vi "Distance Regression Calc.vi"(10 "Numeric in":i32, 11 "Y":dbl) -> (3 "Distance":ext)   [LabVIEW 2025]
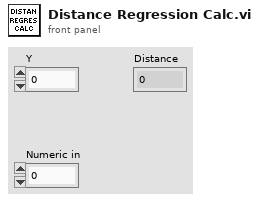
[diagram p1: front panel]
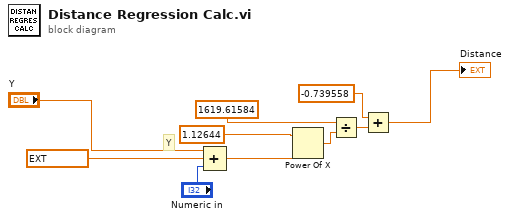
[diagram p0: block diagram]
diagram:
  # "Y"
  n1 = Compound Arithmetic op=unknown("Y", ext -713.92428 ("y"), "Numeric in") -> (w8:ext)
  n2 = Power Of X(1:w8, 2:1.12644 ("y")) -> (0:w3:ext)
  n3 = Divide(x=1619.61584, y=w3) -> (x/y=w5:ext)
  n4 = Add(x=-0.739558, y=w5) -> (x+y=→"Distance":ext)
